vi "SetPFDisplay.vi"(9 "数组":bool[](array[boolean]), 10 "索引 (行)":i32, 11 "TEST 2":refnum<vi>) -> (2 "字符串":string, 3 "引用输出":refnum<vi>)   [LabVIEW 2018]
uses:
  <vilib>/Utility/miscctls.llb/LVRowAndColumnTypeDef.ctl
panel:
  in  "TEST":i32(listbox)
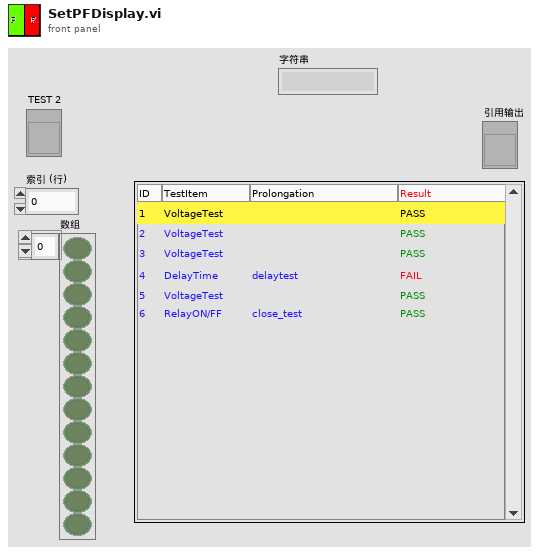
[diagram p1: front panel]
types:
  T1 = typedef "LVRowAndColumnTypeDef.ctl" = cluster{"Row":i32, "Column":i32}
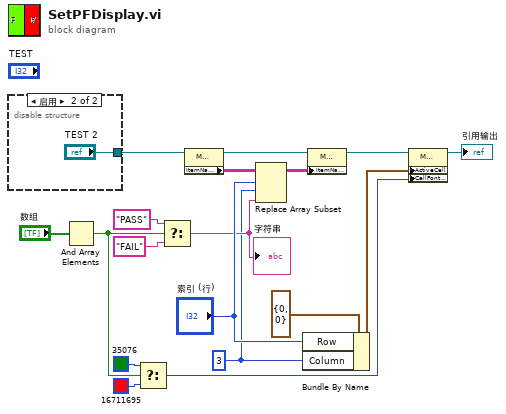
[diagram p0: block diagram]
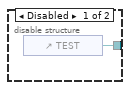
[diagram p2: hidden frame]
diagram:
  w1 = 3 ("禁用的索引 (列)")
  n1 = disable-structure shown="启用" {
    disable-tunnel: [w19 "TEST 2"] -> w17
    frame Disabled {
      n2 = control-ref of="TEST"() -> (w19:refnum<vi>)
    }
    frame Enabled {
    }
  }
  n3 = And Array Elements(Boolean array="数组") -> (logical AND=w3:bool)
  n4 = Select(t=u32 35076, s=w3, f=u32 16711695) -> (s? t:f=w2:u32)
  n5 = Select(t="PASS", s=w3, f="FAIL") -> (s? t:f=w11:string)
  "字符串" <- w11
  n6 = property on="属性节点" class="MCListbox (严格)"(reference=w17) -> (reference out=w9:refnum<vi>, "ItemNames"=w8:string[][])  [unwired: 1 in, 1 out]
  n7 = Replace Array Subset(array=w8, new element=w11, index (row)="索引 (行)", index (col)=w1) -> (w10:string[][])
  n8 = Bundle By Name(cluster=T1 {"Row"=0, "Column"=0} ("活动单元格:活动单元格"), "Row"="索引 (行)", "Column"=w1) -> (w15:T1)
  n9 = property on="属性节点" class="MCListbox (严格)"(reference=w9, "ItemNames"=w10) -> (reference out=w7:refnum<vi>)  [unwired: 1 in, 1 out]
  n10 = property class="MCListbox (严格)"(reference=w7, "ActiveCell"=w15, "CellFontColor"=w2) -> (reference out=→"引用输出":refnum<vi>)  [unwired: 1 in, 1 out]
